vi "Inverse Time Curves (Formula, Definite Reset).vi"(6 "operate time compensation":cluster{"G/Gs":dbl, "compensation [s]":dbl}[](array[cluster]), 7 "GD (25)":u16=25, 8 "error in (no error)":errorcluster, 9 "reset delay (0 s)":dbl, 10 "time multiplier setting (1)":dbl=1.0, 11 "operate time parameters":T1={"A [s]"=1.0, "B [s]"=1.0, "alpha"=1.0, "K2 [s]"=1.0, "K1 [s]"=1.0, "K3 [s]"=1.0}) -> (0 "error out":errorcluster, 2 "memory size":u16, 3 "memory initial values":fxp<+,51,51>[](array[numeric]), 4 "curve data":cluster{"G/Gs":dbl[], "times [s]":dbl[]})   [LabVIEW 2014, in "NI_EP_Protection.lvlib"]
doc: "Generates memory initial values and memory size, which contain the information of the inverse time curves, for the FPGA Inverse Time Delay VI to use. You can compensate for the processing delay of the input energizing quantity under a specific G/Gs to achieve higher operate time accuracy."
uses:
  <vilib>/addons/Electrical Power/Protection/NI_EP_Protection.lvlib
  <vilib>/addons/Electrical Power/Protection/Inverse Time Delay/subVIs/ep_Operate Time.ctl
  <vilib>/addons/Electrical Power/Protection/Inverse Time Delay/subVIs/ep_Curve Parameters.ctl
  <vilib>/addons/Electrical Power/Protection/Inverse Time Delay/subVIs/ep_Reset Time.ctl
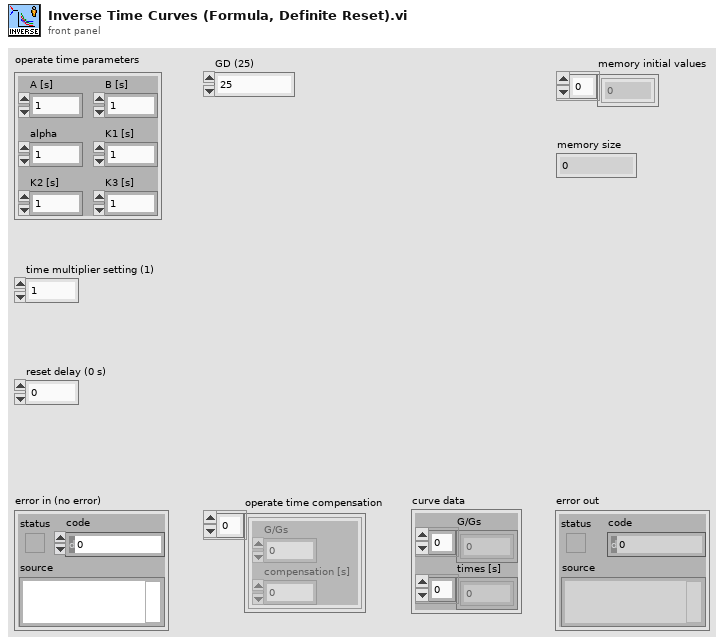
[diagram p1: front panel]
types:
  T1 = typedef "NI_EP_Protection.lvlib/ep_Operate Time.ctl" = cluster{"A [s]":dbl, "B [s]":dbl, "alpha":dbl, "K2 [s]":dbl, "K1 [s]":dbl, "K3 [s]":dbl}
  T2 = typedef "NI_EP_Protection.lvlib/ep_Curve Parameters.ctl" = cluster{"operate time parameters":T1, "reset time parameters":T3}
  T3 = typedef "NI_EP_Protection.lvlib/ep_Reset Time.ctl" = cluster{"tr [s]":dbl, "alpha":dbl}
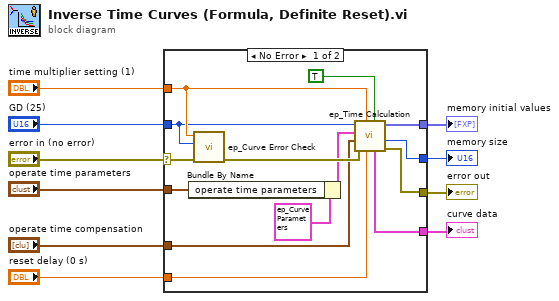
[diagram p0: block diagram]
diagram:
  n1 = case shown="No Error" "error in (no error)" {
    selector: "error in (no error)" -> [w23 w25]
    tunnel: "GD (25)" -> [w22 _]
    tunnel: "time multiplier setting (1)" -> [w24 _]
    tunnel: "operate time parameters" -> [w12 _]
    tunnel: [w19 _] -> w8
    tunnel: [w20 _] -> w7
    tunnel: [w18 w25] -> w5
    tunnel: [w17 _] -> w4
    tunnel: "reset delay (0 s)" -> [w16 _]
    tunnel: "operate time compensation" -> [w11 _]
    frame No Error {
      n2 = Bundle By Name(cluster=T2 {"operate time parameters"={"A [s]"=1.0, "B [s]"=1.0, "alpha"=1.0, "K2 [s]"=1.0, "K1 [s]"=1.0, "K3 [s]"=1.0}, "reset time parameters"={"tr [s]"=1.0, "alpha"=1.0}} ("curve parameters"), "operate time parameters"=w12) -> (w13:T2)
      n3 = call <vilib>:"ep_Curve Error Check.vi"("error in (no error)"=w23, "GD"=w22, "time dial"=w24) -> ("error out"=w21:errorcluster)  [unwired: 8 in]
      n4 = call <vilib>:"ep_Time Calculation.vi"("definite reset? (F)"=TRUE, "reset delay [s]"=w16, "time dial"=w24, "error in (no error)"=w21, "operate time compensation"=w11, "curve parameters"=w13, "GD"=w22) -> ("error out"=w18:errorcluster, "memory size"=w20:u16, "memory initial values"=w19:fxp<+,51,51>[], "curve data"=w17:cluster{"G/Gs":dbl[], "times":dbl[]})  [unwired: 1 in]
    }
    frame Error {
    }
  }
  "memory initial values" <- w8
  "memory size" <- w7
  "error out" <- w5
  "curve data" <- w4
